vi "set_LM_IDs.vi"(8 "error in (no error)":errorcluster caption="错误输入（无错误）", 10 "LM IDs":cluster{"LM ID -":T1, "LM ID +":T1}[](array[cluster]) {"LM ID +" items=["none", "S1", "S2", "S3"]; "LM ID -" items=["none", "S1", "S2", "S3"]}, 11 "MotorSystem 输入":refnum<class "MotorSystem.lvclass">) -> (0 "error out":errorcluster caption="错误输出", 3 "MotorSystem 输出":refnum<class "MotorSystem.lvclass">)   [LabVIEW 2016, in "MotionControl.lvlib" / "MotorSystem.lvclass"]
uses:
  <userlib>/MotionControl/MotorSystem/MotorSystem.lvclass
  <userlib>/MotionControl/LimitSwitch/LM_ID.ctl
  <userlib>/MotionControl/MotorSystem/MotorSystem.lvclass/MotorSystem.ctl
  <userlib>/MotionControl/OneMotion/OneMotion.lvclass/OneMotion.ctl
  <userlib>/MotionControl/LimitSwitch/LimitSwitch.lvclass/LimitSwitch.ctl
  <userlib>/MotionControl/OneMotion/OneMotion.lvclass
  <userlib>/MotionControl/LimitSwitch/LimitSwitch.lvclass
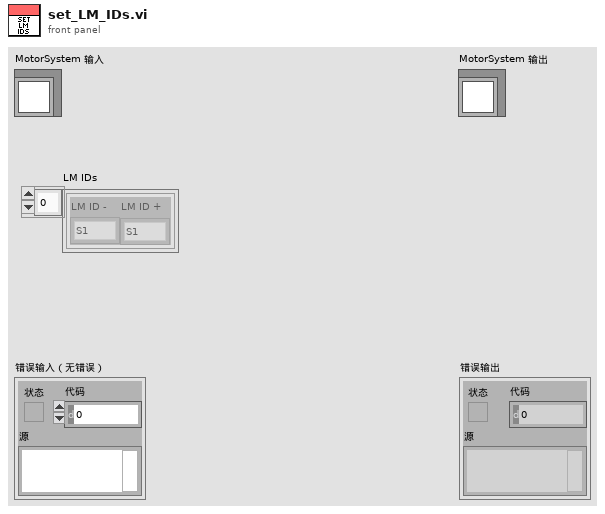
[diagram p1: front panel]
types:
  T1 = typedef "MotionControl.lvlib/LimitSwitch.lvclass/LM_ID.ctl" = i32
  T2 = typedef "MotionControl.lvlib/MotorSystem.lvclass/MotionCluster.ctl" = cluster{"OneMotion.lvclass":refnum<class "OneMotion.lvclass">, "connected?":bool, "default enabled?":bool, "enabled?":bool}
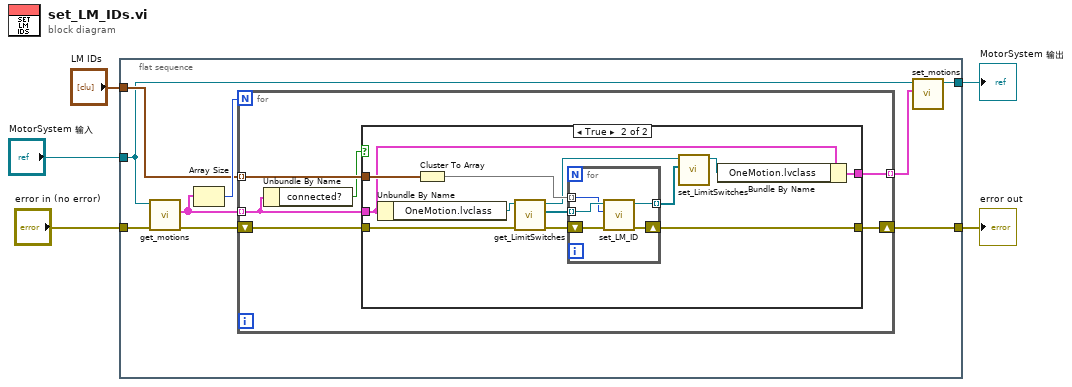
[diagram p0: block diagram]
diagram:
  n1 = flat-sequence {
    tunnel: [w10] -> w5
    tunnel: [w6] -> w3
    tunnel: "MotorSystem 输入" -> [w7]
    tunnel: "error in (no error)" -> [w12]
    tunnel: "LM IDs" -> [w9]
    frame #0 {
      n2 = call <userlib>:"get_motions.vi"("error in (no error)"=w12, "MotorSystem输入"=w7) -> ("error out"=w11:errorcluster, "motions"=w13:T2[])  [unwired: 7 in, 1 out]
      n3 = Array Size(array=w13) -> (size(s)=w14:i32)
      n4 = for {
        N: w14 -> [_]
        tunnel: w13 -> [w16] mode=indexing
        shift-right: [w19] -> w10
        shift-left: w11 -> [w20]
        tunnel: w9 -> [w18] mode=indexing
        tunnel: [w17] -> w8 mode=indexing
        n5 = Unbundle By Name(w16) -> ("connected?"=w15:bool)
        n6 = case shown="True" w15 {
          tunnel: w20 -> [w22 w33]
          tunnel: [w22 w30] -> w19
          tunnel: w18 -> [_ w29]
          tunnel: w16 -> [w21 w26]
          tunnel: [w21 w23] -> w17
          frame False {
          }
          frame True {
            n7 = Unbundle By Name(w26) -> ("OneMotion.lvclass"=w34:refnum<class "OneMotion.lvclass">)
            n8 = Cluster To Array(cluster=w29) -> (array=w28:T1[])
            n9 = call <userlib>:"get_LimitSwitches.vi"("error in (no error)"=w33, "OneMotion输入"=w34) -> ("error out"=w32:errorcluster, "LimitSwitches"=w31:refnum<class "LimitSwitch.lvclass">[], "OneMotion输出"=w25:refnum<class "OneMotion.lvclass">)  [unwired: 7 in]
            n10 = for {
              tunnel: w31 -> [w38] mode=indexing
              shift-right: [w37] -> w30
              shift-left: w32 -> [w39]
              tunnel: w28 -> [w36] mode=indexing
              tunnel: [w35] -> w27 mode=indexing
              n11 = call <userlib>:"set_LM_ID.vi"("error in (no error)"=w39, "LM ID"=w36, "LimitSwitch输入"=w38) -> ("error out"=w37:errorcluster, "LimitSwitch输出"=w35:refnum<class "LimitSwitch.lvclass">)  [unwired: 7 in]
            }
            n12 = call <userlib>:"set_LimitSwitches.vi"("LimitSwitches"=w27, "OneMotion输入"=w25) -> ("OneMotion输出"=w24:refnum<class "OneMotion.lvclass">)  [unwired: 8 in, 1 out]
            n13 = Bundle By Name(cluster=w26, "OneMotion.lvclass"=w24) -> (w23:T2)
          }
        }
      }
      n14 = call <userlib>:"set_motions.vi"("motions"=w8, "MotorSystem输入"=w7) -> ("MotorSystem输出"=w6:refnum<class "MotorSystem.lvclass">)  [unwired: 8 in, 1 out]
    }
  }
  "error out" <- w5
  "MotorSystem 输出" <- w3
